vi "Measure.vi"(10 "measurementservice_DMMConfigResponse_Data":T1, 11 "DMMSession":refnum<k15>) -> (0 "error out":errorcluster, 2 "Measurements":dbl[](array[numeric]))   [LabVIEW 2019, in "ctet_dmm User Library.lvlib"]
uses:
  ctet_dmm User Library.lvlib
  Servers/ctet_dmm/ctet_dmm Class/RPC Messages/measurementservice_DMMConfigResponse/measurementservice_DMMConfigResponse_Data.ctl
  Servers/ctet_dmm/ctet_dmm Class/RPC Messages/measurementservice_ErrorOut/measurementservice_ErrorOut_Data.ctl
  Servers/ctet_dmm/ctet_dmm Class/ctet_dmm.lvclass
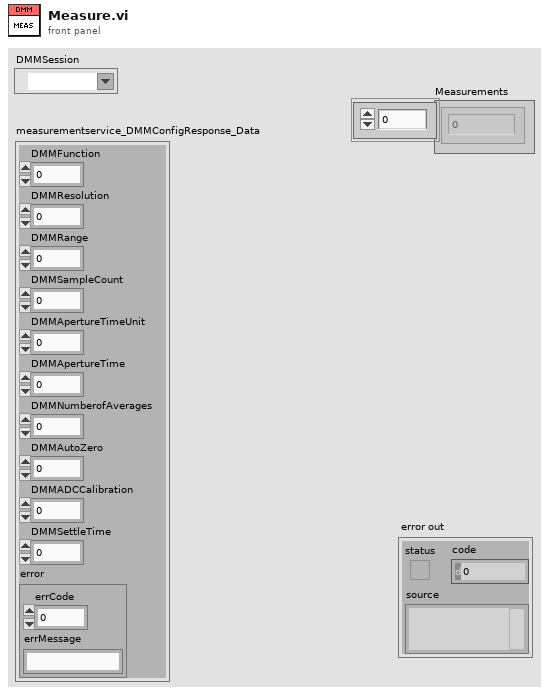
[diagram p1: front panel]
types:
  T1 = typedef "ctet_dmm.lvlib/ctet_dmm.lvclass/measurementservice_DMMConfigResponse_Data.ctl" = cluster{"DMMFunction":i64, "DMMResolution":dbl, "DMMRange":dbl, "DMMSampleCount":i64, "DMMApertureTimeUnit":i64, "DMMApertureTime":dbl, "DMMNumberofAverages":i64, "DMMAutoZero":i64, "DMMADCCalibration":i64, "DMMSettleTime":dbl, "error":T2}
  T2 = typedef "ctet_dmm.lvlib/ctet_dmm.lvclass/measurementservice_ErrorOut_Data.ctl" = cluster{"errCode":i64, "errMessage":string}
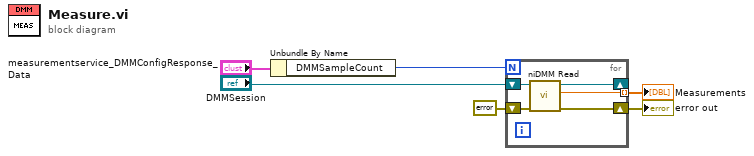
[diagram p0: block diagram]
diagram:
  n1 = Unbundle By Name("measurementservice_DMMConfigResponse_Data") -> ("DMMSampleCount"=w4:i64)
  n2 = for {
    N: w4 -> [_]
    shift-right: [w10] -> w6
    shift-left: errorcluster {"status"=FALSE, "code"=0, "source"=""} ("error out") -> [w9]
    shift-right: [w11] -> _
    shift-left: "DMMSession" -> [w8]
    tunnel: [w7] -> w1 mode=indexing
    n3 = call <instrlib>:"niDMM Read.vi"("error in (no error)"=w9, "instrument handle"=w8) -> ("error out"=w10:errorcluster, "Measurement"=w7:dbl, "instrument handle out"=w11:refnum<k15>)  [unwired: 7 in]
  }
  "error out" <- w6
  "Measurements" <- w1
